vi "CalculateEndTimeSubVI.vi"(10 "Wait Time (Seconds)":dbl=4.0, 11 "Current Time (Seconds)":dbl) -> (3 "End Time (Seconds)":dbl)   [LabVIEW 2019]
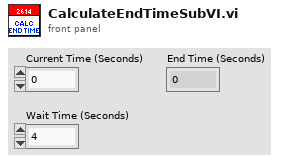
[diagram p1: front panel]
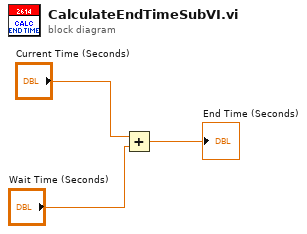
[diagram p0: block diagram]
diagram:
  n1 = Add(x="Current Time (Seconds)", y="Wait Time (Seconds)") -> (x+y=→"End Time (Seconds)":dbl)
